vi "File Path to Hyperlink.vi"(8 "error in (no error)":errorcluster, 11 "File Path":path) -> (0 "error out":errorcluster, 3 "Hyperlink":string)   [LabVIEW 2015]
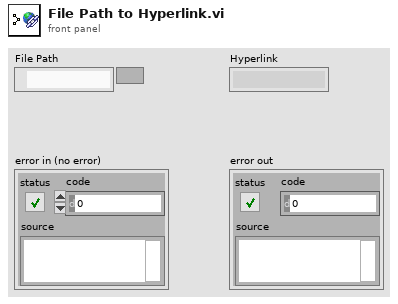
[diagram p1: front panel]
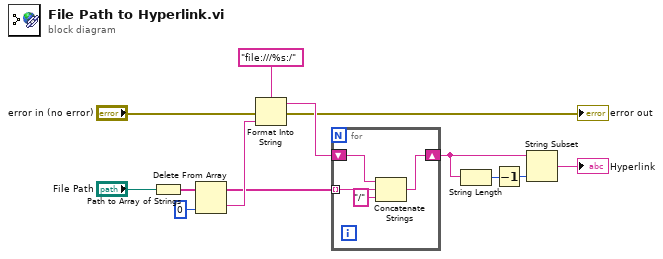
[diagram p0: block diagram]
diagram:
  n1 = Path to Array of Strings(0:"File Path") -> (2:w8:string[])  [unwired: 1 out]
  n2 = Delete From Array(array=w8, index=0) -> (deleted portion=w11:string, array with subset deleted=w10:string[])  [unwired: 1 in]
  n3 = Format Into String(format string="file:///%s:/", error in="error in (no error)", w11) -> (resulting string=w12:string, error out=→"error out":errorcluster)  [unwired: 1 in]
  n4 = for {
    tunnel: w10 -> [w17] mode=indexing
    shift-right: [w14] -> w4
    shift-left: w12 -> [w16]
    n5 = Concatenate Strings(w16, w17, "/" ("string")) -> (w14:string)
  }
  n6 = String Length(string=w4) -> (length=w5:i32)
  n7 = Decrement(x=w5) -> (x-1=w7:i32)
  n8 = String Subset(string=w4, length (rest)=w7) -> (substring=→"Hyperlink":string)  [unwired: 1 in]
